vi "test.vi"   [LabVIEW 2012]
uses:
  <resource>/objmgr/daqmx.rc
  <vilib>/Waveform/DWDTOps.llb/Digital Pattern Generator (Single Value).vi
  <vilib>/Waveform/DWDTOps.llb/DWDT Digital Size.vi
  <vilib>/DAQmx/write.llb/DAQmx Write (Digital Wfm 1Chan NSamp).vi
  <vilib>/DAQmx/configure/timing.llb/DAQmx Timing (Sample Clock).vi
  <vilib>/DAQmx/create/channels.llb/DAQmx Create Channel (DO-Digital Output).vi
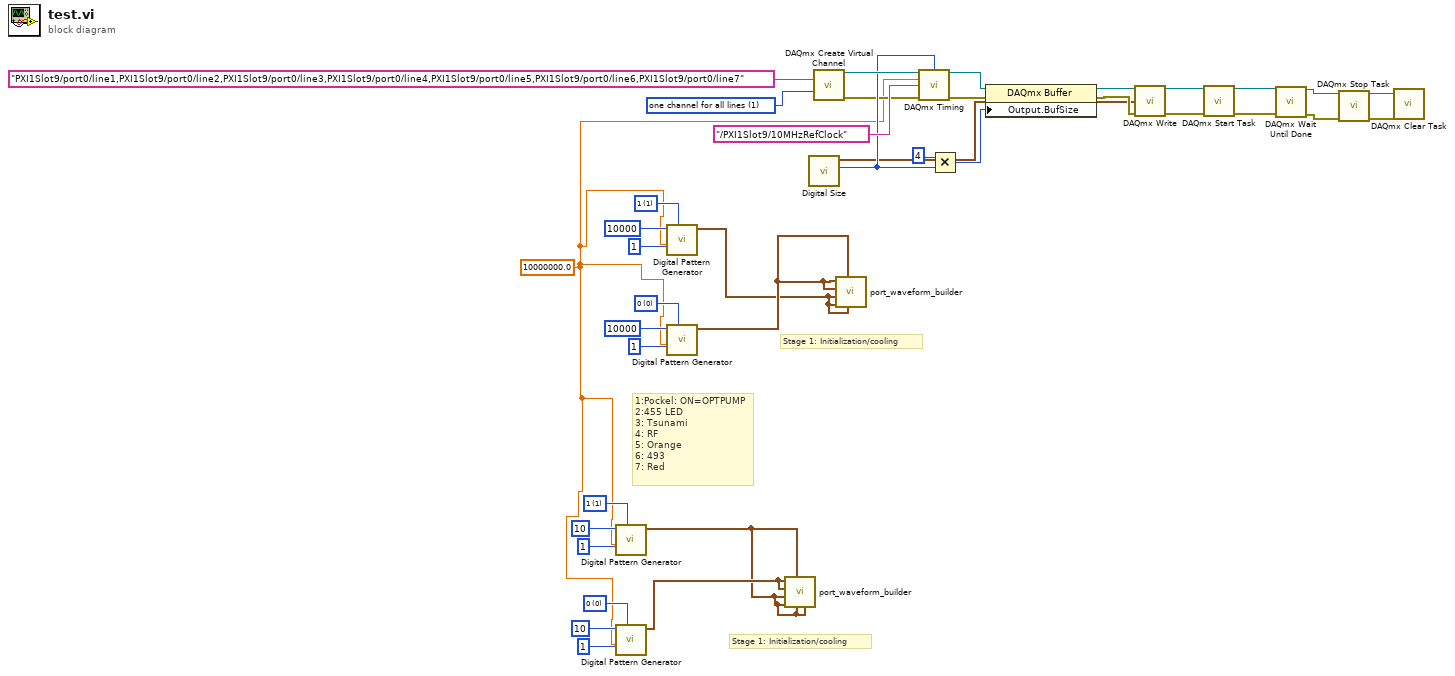
[diagram p0: block diagram]
diagram:
  w6 = u8 0 items=["0", "1", "Z", "L", "H", "X", "T", "V"] ("value")
  w9 = u8 1 items=["0", "1", "Z", "L", "H", "X", "T", "V"] ("value")
  w14 = u8 0 items=["0", "1", "Z", "L", "H", "X", "T", "V"] ("value")
  w17 = u8 1 items=["0", "1", "Z", "L", "H", "X", "T", "V"] ("value")
  w29 = 1 items=["one channel for each line", "one channel for all lines"] ("line grouping")
  w2 = 10000000.0 ("rate")
  # "Stage 1: Initialization/cooling"
  # "Stage 1: Initialization/cooling"
  # "1:Pockel: ON=OPTPUMP\n2:455 LED\n3: Tsunami\n4: RF\n5: Orange\n6: 493\n7: Red"
  n1 = call-poly <vilib>:"Digital Pattern Generator.vi"("value"=w9, "sample rate"=w2, "number of signals"=u32 1, "number of samples"=u32 10) -> ("digital waveform"=w1:digitalwaveform)  [unwired: 6 in, 1 out]
  n2 = call-poly <vilib>:"Digital Pattern Generator.vi"("value"=w6, "sample rate"=w2, "number of signals"=u32 1, "number of samples"=u32 10) -> ("digital waveform"=w3:digitalwaveform)  [unwired: 6 in, 1 out]
  n3 = call-poly <vilib>:"Digital Pattern Generator.vi"("value"=w17, "sample rate"=w2, "number of signals"=u32 1, "number of samples"=u32 10000) -> ("digital waveform"=w10:digitalwaveform)  [unwired: 6 in, 1 out]
  n4 = call-poly <vilib>:"Digital Pattern Generator.vi"("value"=w14, "sample rate"=w2, "number of signals"=u32 1, "number of samples"=u32 10000) -> ("digital waveform"=w11:digitalwaveform)  [unwired: 6 in, 1 out]
  n5 = call "port_waveform_builder.vi"("Line 7"=w1, "Line 6"=w1, "Line 1"=w1, "Line 5"=w1, "Line 4"=w1, "Line 3"=w3, "Line 2"=w3) -> ()  [unwired: 4 in, 1 out]
  n6 = call-poly <vilib>:"DAQmx Create Virtual Channel.vi"("lines"=tag "PXI1Slot9/port0/line1,PXI1Slot9/port0/line2,PXI1Slot9/port0/line3,PXI1Slot9/port0/line4,PXI1Slot9/port0/line5,PXI1Slot9/port0/line6,PXI1Slot9/port0/line7", "line grouping"=w29) -> ("task out"=w31:refnum<k21>, "error out"=w27:errorcluster)  [unwired: 12 in]
  n7 = call "port_waveform_builder.vi"("Line 6"=w10, "Line 1"=w11, "Line 5"=w10, "Line 4"=w10, "Line 3"=w11, "Line 2"=w11) -> ()  [unwired: 5 in, 1 out]
  n8 = call-poly <vilib>:"Digital Size.vi"("digital waveform in"=w18) -> ("number of samples"=w30:i32)  [unwired: 7 in, 3 out]
  n9 = call-poly <vilib>:"DAQmx Timing.vi"("task/channels in"=w31, "samples per channel"=w30, "rate"=w2, "source"=tag "/PXI1Slot9/10MHzRefClock", "error in"=w27) -> ("task out"=w37:refnum<k21>, "error out"=w36:errorcluster)  [unwired: 9 in]
  n10 = Multiply(x=4, y=w30) -> (x*y=w35:i32)
  n11 = property class="DAQmx Buffer"(reference=w37, error in=w36, "Output.BufSize"=w35) -> (reference out=w33:refnum<k21>, error out=w26:errorcluster)
  n12 = call-poly <vilib>:"DAQmx Write.vi"("task/channels in"=w33, "error in"=w26) -> ("task out"=w32:refnum<k21>, "data"=w18:digitalwaveform, "error out"=w25:errorcluster)  [unwired: 10 in, 1 out]
  n13 = call <vilib>:"DAQmx Start Task.vi"("task/channels in"=w32, "error in"=w25) -> ("task out"=w23:refnum<k21>, "error out"=w24:errorcluster)  [unwired: 12 in]
  n14 = call <vilib>:"DAQmx Wait Until Done.vi"("task/channels in"=w23, "error in"=w24) -> ("task out"=w22:refnum<k21>, "error out"=w20:errorcluster)  [unwired: 12 in]
  n15 = call <vilib>:"DAQmx Stop Task.vi"("task/channels in"=w22, "error in"=w20) -> ("task out"=w21:refnum<k21>, "error out"=w19:errorcluster)  [unwired: 12 in]
  n16 = call <vilib>:"DAQmx Clear Task.vi"("task in"=w21, "error in"=w19) -> ()  [unwired: 13 in, 1 out]
